vi "azcamtool.vi"() -> ()   [LabVIEW 2014]
doc: "AzCamTool"
uses:
  globals/AzCamGlobals.vi
  globals/DetectorGlobals.vi
panel:
  in  "Image Type":u16(ring) items=["zero", "object", "flat", "dark", "LED", "Fe55"]
  in  "Exposure Time":dbl=1.0 min=0.0 format="%<%S%3u>t"
  out "Image Filename":string
  out "StatusBar":string
  in  "TestImage":bool=TRUE caption="Test Image"
  in  "Image Title":string
  out "rowbin":u32=1 min=1 max=99 step=1
  out "colbin":u32=1 min=1 max=99 step=1
  out "progress":dbl(slide) scale=0.0..100.0 scale format="%.1e"
  out "CamTemp":sgl=-999.9 format="%.1f"
  out "DewTemp":sgl=-999.9 format="%.1f"
  out "SequenceCount":string caption="Seq. Count"
  out "Current Exposure Time":dbl caption="Exposure Time" min=0.0 format="%<%S%3u>t"
  out "ImageTypeName":string caption="ImageType"
  in  "Abort":bool
  in  "Reset":bool
  in  "Pause":bool
  in  "Resume":bool
  in  "Readout":bool
  out "CurrentImageTitle":string caption="ImageTitle"
  out "Error":bool
  in  "Expose":bool
  in  "Sequence":bool
  in  "Num Seq.":u16=1 min=1 step=1
  in  "Detector":bool
  in  "FilenameBut":bool caption="Filename"
  in  "Preferences":bool
  out "Test Image":bool
  # "Control"
  # "Status"
  # "Binning"
  # "Exposure Status"
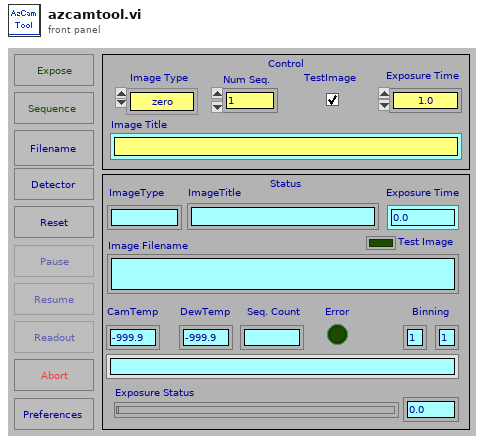
[diagram p1: front panel]
types:
  T1 = enum16{"Standard", "Buffered", "CRLF", "Immediate"}
  T2 = enum16{"Start", "Stop", "Abort", "Pause", "SetExposureTime", "GetExposureTimeRemaining", "Resume", "Readout", "GetExposureTime", "GetTotalPixels", "GetPixelsRemaining"}
  T3 = enum16{"Start", "Stop", "Abort", "Pause", "SetExposureTime", "GetExposureTimeRemaining", "Resume", "Readout", "GetExposureTime"}
  T4 = enum16{"Start", "Stop", "Abort", "Pause", "SetExposureTime", "GetExposureTimeRemaining", "Resume"}
  T5 = enum16{"Start", "Stop", "Abort", "Pause", "SetExposureTime", "GetExposureTimeRemaining", "Resume", "Readout"}
  T6 = enum32{"invalid app kind", "Development System", "Run Time System", "Student Edition", "Embedded LabVIEW", "Evaluation", "Custom"}
  T7 = enum32{"invalid OS target", "Mac OS", "Windows 3.1", "Windows 95/NT", "Solaris 1", "Solaris 2", "HP-UX", "PowerMAX", "Linux", "Irix", "Rhapsody", "BeOS", "AIX", "OSF1", "VxWorks", "PharLap", "Carbon", "RTX", "Windows x64", "Linux x64", "Mac OS X x64"}
  T8 = enum8{"Enabled", "Disabled", "Disabled and Grayed Out"}
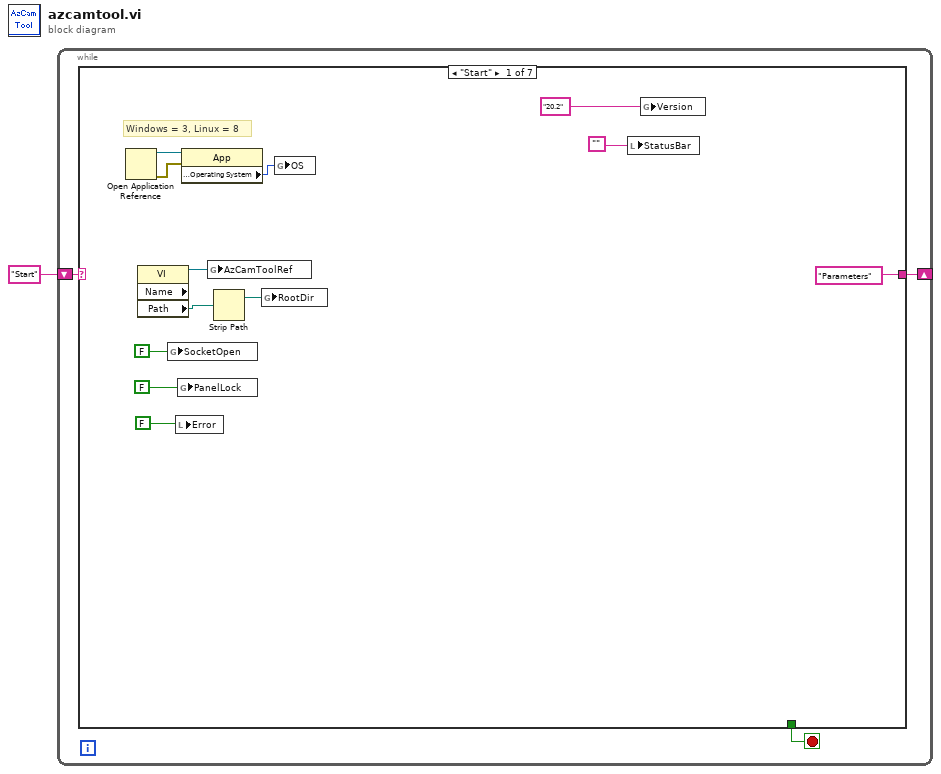
[diagram p0: block diagram]
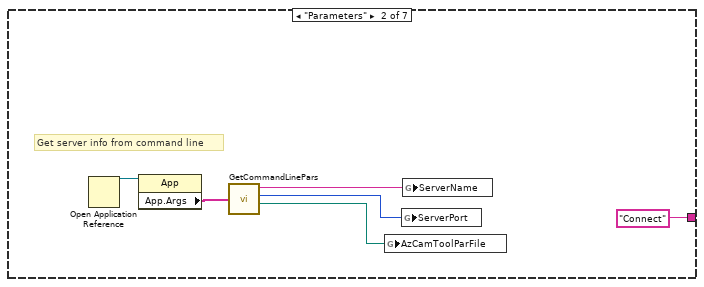
[diagram p2: hidden frame]
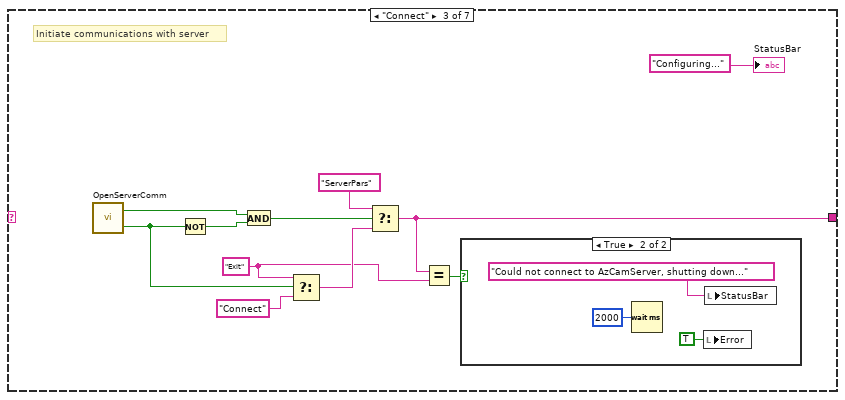
[diagram p3: hidden frame]
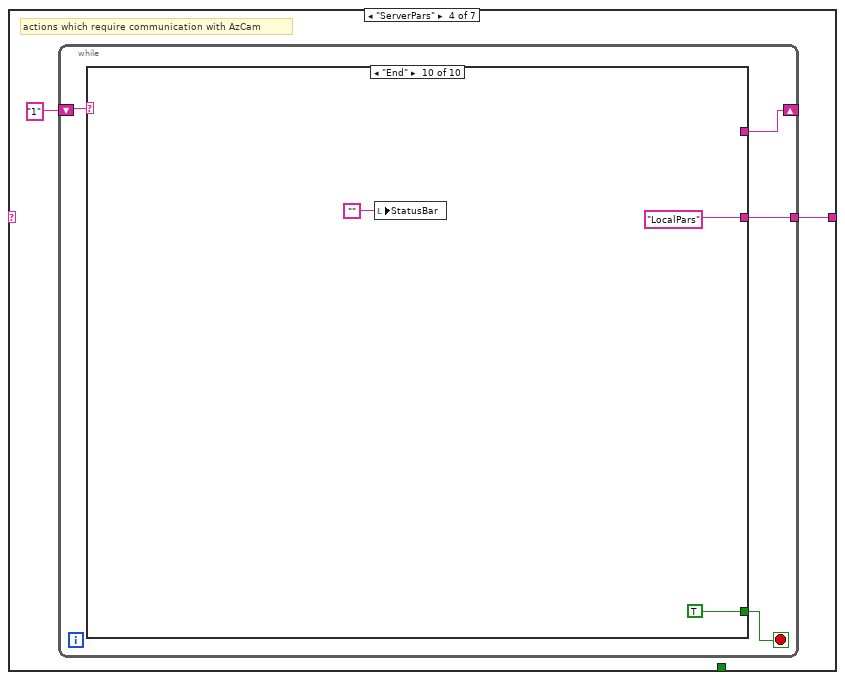
[diagram p5: hidden frame]
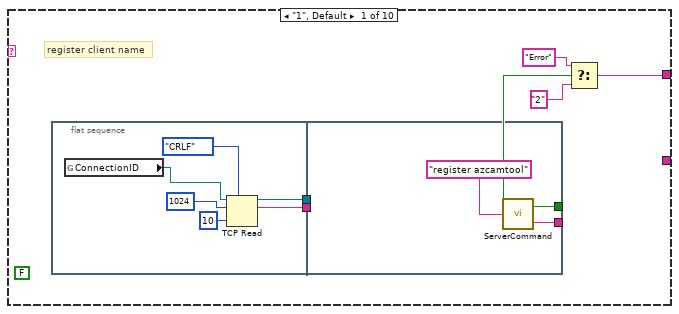
[diagram p6: hidden frame]
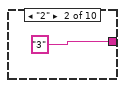
[diagram p7: hidden frame]
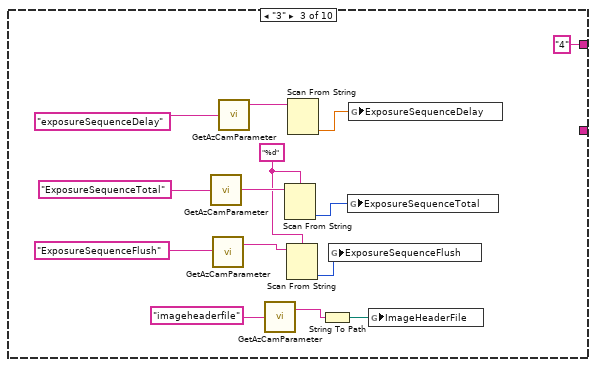
[diagram p8: hidden frame]
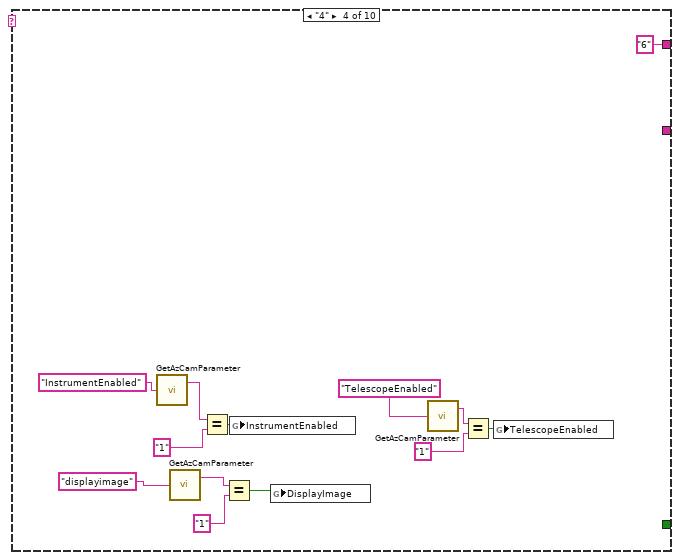
[diagram p9: hidden frame]
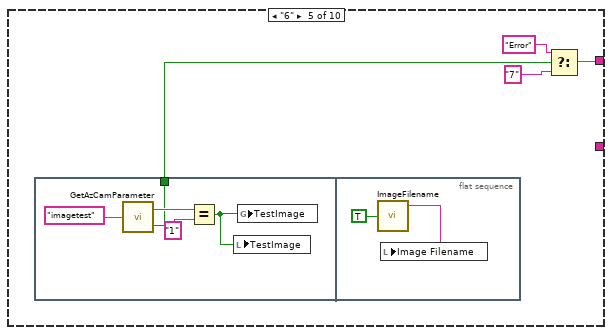
[diagram p10: hidden frame]
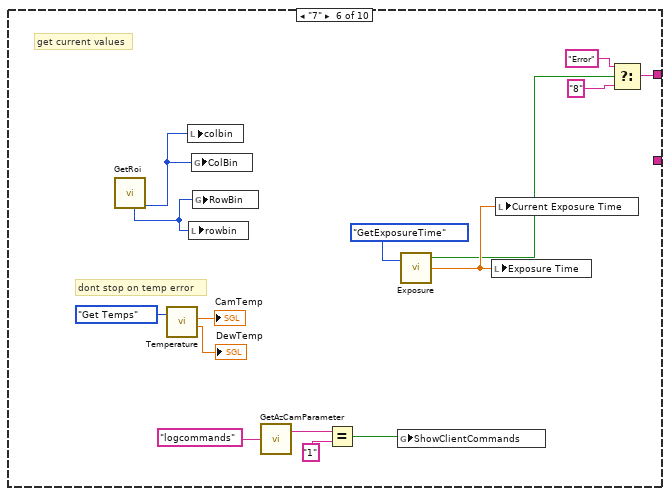
[diagram p11: hidden frame]
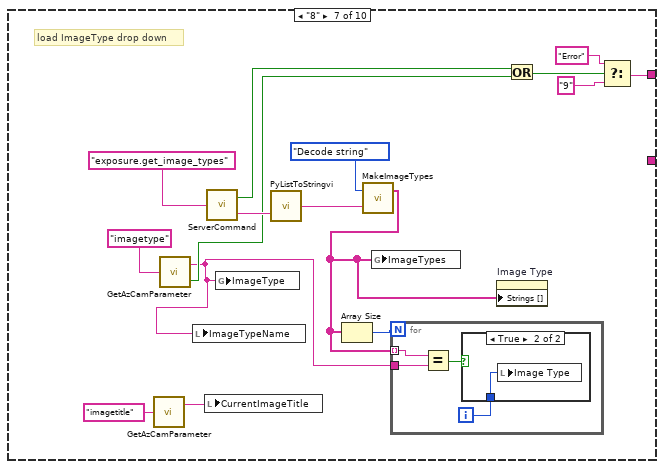
[diagram p12: hidden frame]
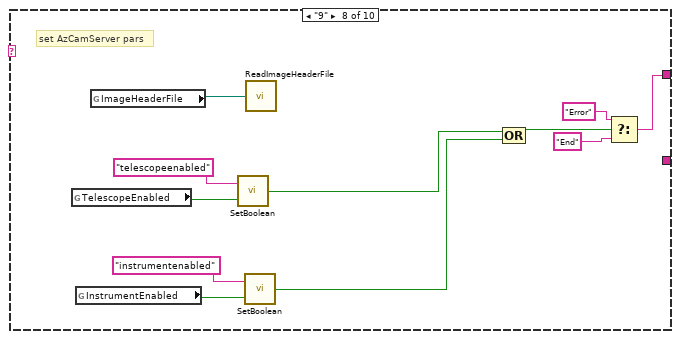
[diagram p14: hidden frame]
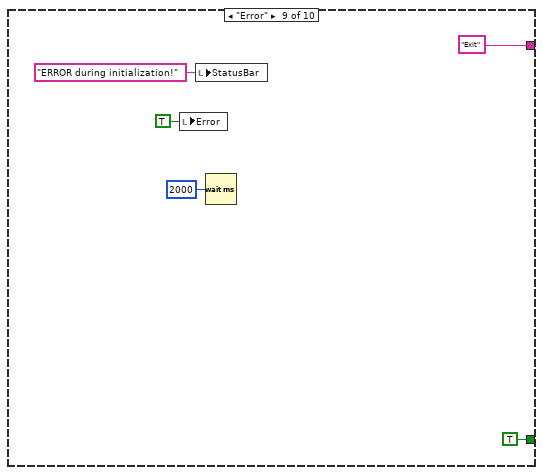
[diagram p15: hidden frame]
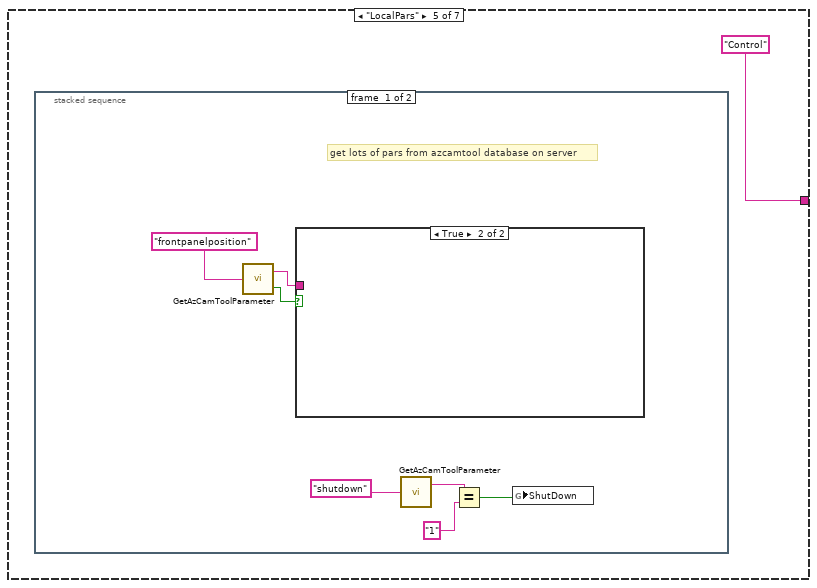
[diagram p16: hidden frame]
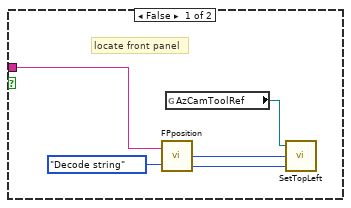
[diagram p17: hidden frame]
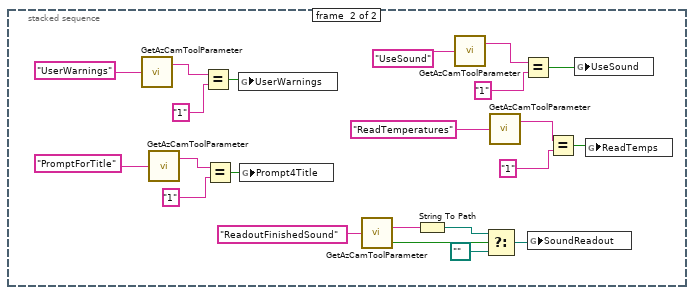
[diagram p18: hidden frame]
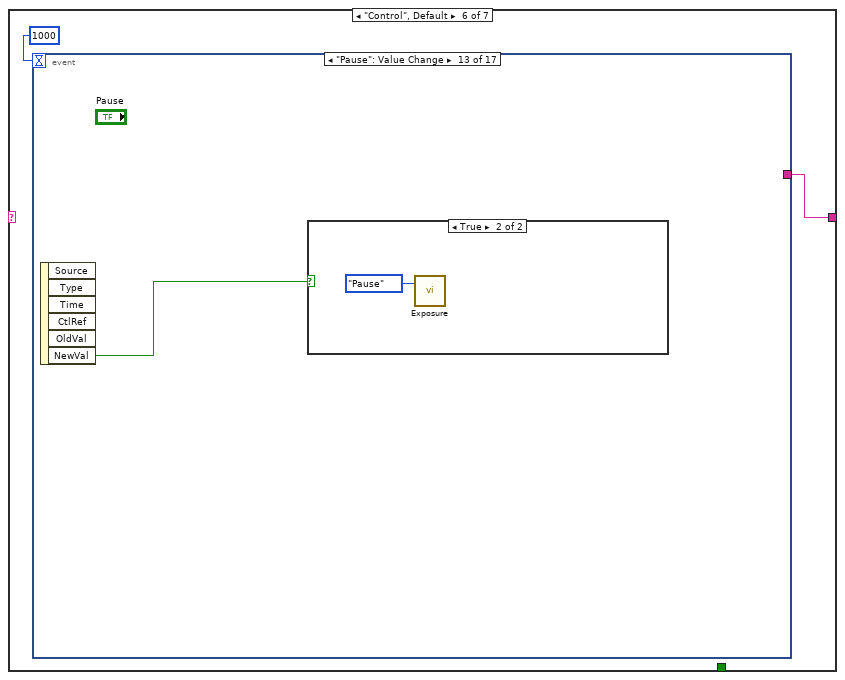
[diagram p19: hidden frame]
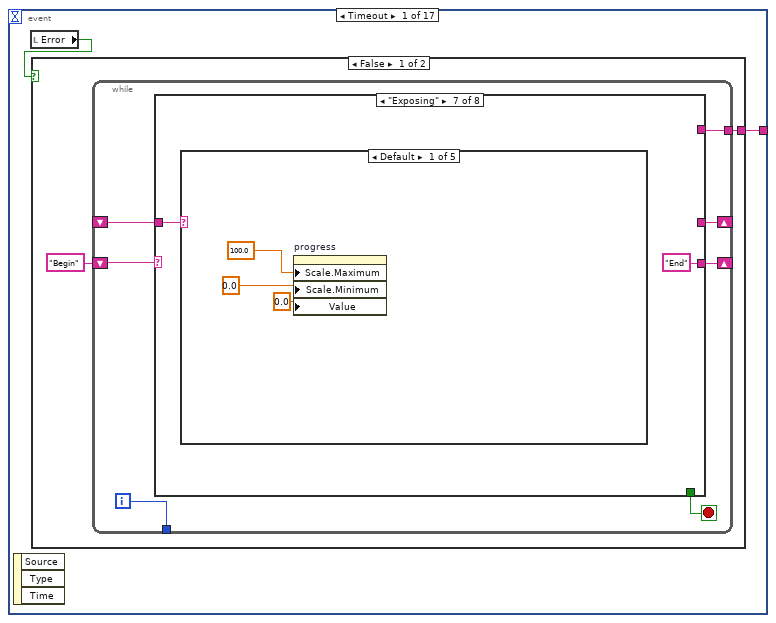
[diagram p20: hidden frame]
diagram:
  n1 = while {
    shift-right: [w2] -> _
    shift-left: "Start" ("Command") -> [w3]
    stop <- w4 stop-if-true
    n2 = case shown="\"Start\"" w3 {
      tunnel: [_ _ _ _ _ _ TRUE] -> w4
      tunnel: ["Parameters" "Connect" ("f") w25 w38 "Control" w188 _] -> w2
      frame "Start" {
        # "Windows = 3, Linux = 8"
        n3 = Open Application Reference() -> (0:w15:errorcluster, 3:w16:refnum<vi>)  [unwired: 4 in]
        n4 = property class="VI" props=["Name", "Path"]() -> (reference out=w7:refnum<vi>, "Path"=w11:path)  [unwired: 2 in, 2 out]
        n5 = global write "AzCamGlobals.vi" "SocketOpen"(FALSE ("SocketOpen")) -> ()
        n6 = local write "Error"(FALSE ("Error")) -> ()
        n7 = global write "AzCamGlobals.vi" "PanelLock"(FALSE ("LockFlag")) -> ()
        n8 = property class="App"(reference=w16, error in=w15) -> ("Application:Target:Operating System"=w13:T7)  [unwired: 2 out]
        n9 = global write "AzCamGlobals.vi" "AzCamToolRef"(w7) -> ()
        n10 = Strip Path(path=w11) -> (stripped path=w9:path)  [unwired: 1 out]
        n11 = global write "AzCamGlobals.vi" "RootDir"(w9) -> ()
        n12 = global write "AzCamGlobals.vi" "OS"(w13) -> ()
        n13 = local write "StatusBar"("") -> ()
        n14 = global write "AzCamGlobals.vi" "Version"("20.2" ("Version Date")) -> ()
      }
      frame "Parameters" {
        # "Get server info from command line"
        n15 = Open Application Reference() -> (3:w20:refnum<vi>)  [unwired: 4 in, 1 out]
        n16 = property class="App"(reference=w20) -> ("App.Args"=w21:string[])  [unwired: 1 in, 2 out]
        n17 = call "GetCommandLinePars.vi"("Command line array"=w21) -> ("Server"=w19:string, "Port"=w18:i32, "AzCamToolParFile"=w17:path)  [unwired: 1 out]
        n18 = global write "AzCamGlobals.vi" "AzCamToolParFile"(w17) -> ()
        n19 = global write "AzCamGlobals.vi" "ServerPort"(w18) -> ()
        n20 = global write "AzCamGlobals.vi" "ServerName"(w19) -> ()
      }
      frame "Connect" {
        w24 = "Exit" ("f")
        # "Initiate communications with server"
        n21 = call "OpenServerComm.vi"() -> ("Connected"=w32:bool, "Quitted"=w26:bool)  [unwired: 1 in]
        n22 = Not(x=w26) -> (.not. x?=w31:bool)
        n23 = And(x=w32, y=w31) -> (x .and. y?=w33:bool)
        n24 = Select(t=w24, s=w26, f="Connect") -> (s? t:f=w28:string)
        n25 = Select(t="ServerPars" ("f"), s=w33, f=w28) -> (s? t:f=w25:string)
        n26 = Equal?(x=w25, y=w24) -> (x = y?=w23:bool)
        n27 = case shown="True" w23 {
          frame False {
          }
          frame True {
            n28 = Wait (ms)(milliseconds to wait=u32 2000) -> ()  [unwired: 1 out]
            n29 = local write "Error"(TRUE ("Error")) -> ()
            n30 = local write "StatusBar"("Could not connect to AzCamServer, shutting down..." ("StatusBar")) -> ()
          }
        }
        "StatusBar" <- "Configuring..." ("Messages")
      }
      frame "ServerPars" {
        # "actions which require communication with AzCam"
        n31 = while {
          tunnel: [w40] -> w38
          shift-right: [w41] -> _
          shift-left: "1" ("key") -> [w42]
          stop <- w39 stop-if-true
          n32 = case shown="\"End\"" w42 {
            tunnel: [w46 "3" ("key") "4" ("key") "6" ("key") w87 w106 w118 w138 _ _] -> w41
            tunnel: [_ _ _ _ _ _ _ _ "Exit" "LocalPars"] -> w40
            tunnel: [_ _ _ _ _ _ _ _ TRUE TRUE] -> w39
            frame "1", Default {
              (unwired) FALSE
              # "register client name"
              n33 = flat-sequence {
                tunnel: [w51] -> w44
                tunnel: [w50] -> w43
                tunnel: [w56] -> _
                tunnel: [w55] -> w45
                tunnel: w44 -> [_]
                tunnel: w43 -> [_]
                frame #0 {
                  n34 = global read "AzCamGlobals.vi" "ConnectionID"() -> (w49:refnum<k5>)
                  n35 = TCP Read(connection ID=w49, bytes to read=1024, 7:T1."CRLF" ("mode (standard)"), 9:10 ("timeout ms (25000)")) -> (connection ID out=w50:refnum<k5>, data out=w51:string)  [unwired: 1 in, 1 out]
                }
                frame #1 {
                  n36 = call "ServerCommand.vi"("Command"="register azcamtool") -> ("Error"=w55:bool, "Reply"=w56:string)
                }
              }
              n37 = Select(t="Error" ("key"), s=w45, f="2" ("key")) -> (s? t:f=w46:string)
            }
            frame "2" {
            }
            frame "3" {
              w67 = "%d" ("format string")
              n38 = call "GetAzCamParameter.vi"("Parameter"="ExposureSequenceTotal") -> ("Value"=w71:string)  [unwired: 1 out]
              n39 = call "GetAzCamParameter.vi"("Parameter"="ExposureSequenceFlush") -> ("Value"=w62:string)  [unwired: 1 out]
              n40 = call "GetAzCamParameter.vi"("Parameter"="exposureSequenceDelay") -> ("Value"=w69:string)  [unwired: 1 out]
              n41 = call "GetAzCamParameter.vi"("Parameter"="imageheaderfile" ("key")) -> ("Value"=w61:string)  [unwired: 1 out]
              n42 = Scan From String(format string=w67, input string=w71) -> (output 1=w65:i32)  [unwired: 3 in, 3 out]
              n43 = Scan From String(format string=w67, input string=w62) -> (output 1=w66:i32)  [unwired: 3 in, 3 out]
              n44 = Scan From String(input string=w69) -> (output 1=w64:dbl)  [unwired: 4 in, 3 out]
              n45 = String To Path(string=w61) -> (path=w63:path)
              n46 = global write "AzCamGlobals.vi" "ExposureSequenceFlush"(w66) -> ()
              n47 = global write "AzCamGlobals.vi" "ExposureSequenceTotal"(w65) -> ()
              n48 = global write "AzCamGlobals.vi" "ExposureSequenceDelay"(w64) -> ()
              n49 = global write "AzCamGlobals.vi" "ImageHeaderFile"(w63) -> ()
            }
            frame "4" {
              n50 = call "GetAzCamParameter.vi"("Parameter"="InstrumentEnabled" ("key")) -> ("Value"=w73:string)  [unwired: 1 out]
              n51 = call "GetAzCamParameter.vi"("Parameter"="displayimage" ("key")) -> ("Value"=w76:string)  [unwired: 1 out]
              n52 = Equal?(x=w73, y="1") -> (x = y?=w81:bool)
              n53 = Equal?(x=w76, y="1") -> (x = y?=w80:bool)
              n54 = global write "AzCamGlobals.vi" "InstrumentEnabled"(w81) -> ()
              n55 = global write "AzCamGlobals.vi" "DisplayImage"(w80) -> ()
              n56 = call "GetAzCamParameter.vi"("Parameter"="TelescopeEnabled" ("key")) -> ("Value"=w77:string)  [unwired: 1 out]
              n57 = Equal?(x=w77, y="1") -> (x = y?=w84:bool)
              n58 = global write "AzCamGlobals.vi" "TelescopeEnabled"(w84) -> ()
            }
            frame "6" {
              n59 = flat-sequence {
                tunnel: [w90] -> w86
                frame #0 {
                  n60 = call "GetAzCamParameter.vi"("Parameter"="imagetest") -> ("Error"=w90:bool, "Value"=w91:string)
                  n61 = Equal?(x=w91, y="1") -> (x = y?=w94:bool)
                  n62 = local write "TestImage"(w94) -> ()
                  n63 = global write "AzCamGlobals.vi" "TestImage"(w94) -> ()
                }
                frame #1 {
                  n64 = call "ImageFilename.vi"("Immediate"=TRUE) -> ("Output Image Filename"=w96:string)  [unwired: 2 out]
                  n65 = local write "Image Filename"(w96) -> ()
                }
              }
              n66 = Select(t="Error" ("key"), s=w86, f="7" ("key")) -> (s? t:f=w87:string)
            }
            frame "7" {
              # "dont stop on temp error"
              # "get current values"
              n67 = call "GetRoi.vi"() -> ("RowBin"=w110:i32, "ColBin"=w111:i32)  [unwired: 1 in, 4 out]
              n68 = call "Temperature.vi"("Action"=enum16{"Set Celsius", "Get Temps"}."Get Temps") -> ("Output2"=→"DewTemp":sgl, "Output1"=→"CamTemp":sgl)  [unwired: 1 in, 3 out]
              n69 = local write "colbin"(w111) -> ()
              n70 = local write "rowbin"(w110) -> ()
              n71 = global write "DetectorGlobals.vi" "ColBin"(w111) -> ()
              n72 = global write "DetectorGlobals.vi" "RowBin"(w110) -> ()
              n73 = call "GetAzCamParameter.vi"("Parameter"="logcommands") -> ("Value"=w98:string)  [unwired: 1 out]
              n74 = Equal?(x=w98, y="1") -> (x = y?=w97:bool)
              n75 = global write "AzCamGlobals.vi" "ShowClientCommands"(w97) -> ()
              n76 = call "Exposure.vi"("Command"=T2."GetExposureTime") -> ("Error"=w101:bool, "float"=w102:dbl)  [unwired: 1 in, 1 out]
              n77 = local write "Exposure Time"(w102) -> ()
              n78 = local write "Current Exposure Time"(w102) -> ()
              n79 = Select(t="Error" ("key"), s=w101, f="8" ("key")) -> (s? t:f=w106:string)
            }
            frame "8" {
              # "load ImageType drop down"
              n80 = call "GetAzCamParameter.vi"("Parameter"="imagetitle") -> ("Value"=w112:string)  [unwired: 1 out]
              n81 = call "GetAzCamParameter.vi"("Parameter"="imagetype") -> ("Error"=w115:bool, "Value"=w114:string)
              n82 = local write "ImageTypeName"(w114) -> ()
              n83 = local write "CurrentImageTitle"(w112) -> ()
              n84 = call "ServerCommand.vi"("Command"="exposure.get_image_types") -> ("Error"=w116:bool, "Reply"=w125:string)
              n85 = global write "AzCamGlobals.vi" "ImageType"(w114) -> ()
              n86 = call "PyListToStringvi.vi"("PythonList"=w125) -> ("String"=w124:string)
              n87 = call "MakeImageTypes.vi"("String In"=w124, "Action"=enum16{"Make string", "Decode string"}."Decode string") -> ("ImageTypes"=w122:string[])  [unwired: 1 out]
              n88 = Array Size(array=w122) -> (size(s)=w123:i32)
              n89 = global write "AzCamGlobals.vi" "ImageTypes"(w122) -> ()
              n90 = for {
                N: w123 -> [_]
                tunnel: w122 -> [w131] mode=indexing
                tunnel: w114 -> [w130]
                i -> [w128]
                n91 = Equal?(x=w131, y=w130) -> (x = y?=w129:bool)
                n92 = case shown="True" w129 {
                  tunnel: w128 -> [_ w132]
                  frame False {
                  }
                  frame True {
                    n93 = local write "Image Type"(w132) -> ()
                  }
                }
              }
              n94 = property on="Image Type" class="Ring (strict)"("Strings []"=w122) -> ()  [unwired: 2 in, 2 out]
              n95 = Or(x=w116, y=w115) -> (x .or. y?=w117:bool)
              n96 = Select(t="Error" ("key"), s=w117, f="9" ("key")) -> (s? t:f=w118:string)
            }
            frame "9" {
              # "set AzCamServer pars"
              n97 = global read "AzCamGlobals.vi" "TelescopeEnabled"() -> (w135:bool)
              n98 = global read "AzCamGlobals.vi" "InstrumentEnabled"() -> (w134:bool)
              n99 = global read "AzCamGlobals.vi" "ImageHeaderFile"() -> (w133:path)
              n100 = call "SetBoolean.vi"("Boolean"=w135, "Attribute"="telescopeenabled" ("Command")) -> ("Error"=w137:bool)
              n101 = call "SetBoolean.vi"("Boolean"=w134, "Attribute"="instrumentenabled" ("Command")) -> ("Error"=w136:bool)
              n102 = call "ReadImageHeaderFile.vi"("ImageHeaderFile"=w133) -> ()  [unwired: 1 in]
              n103 = Compound Arithmetic op=OR(w137, w136) -> (w139:bool)
              n104 = Select(t="Error" ("key"), s=w139, f="End" ("key")) -> (s? t:f=w138:string)
            }
            frame "Error" {
              n105 = local write "Error"(TRUE ("Error")) -> ()
              n106 = local write "StatusBar"("ERROR during initialization!" ("StatusBar")) -> ()
              n107 = Wait (ms)(milliseconds to wait=u32 2000) -> ()  [unwired: 1 out]
            }
            frame "End" {
              n108 = local write "StatusBar"("") -> ()
            }
          }
        }
      }
      frame "LocalPars" {
        n109 = stacked-sequence {
          frame #0 {
            # "get lots of pars from azcamtool database on server"
            n110 = call "GetAzCamToolParameter.vi"("Parameter"="frontpanelposition" ("key")) -> ("Error"=w158:bool, "Value"=w159:string)
            n111 = case shown="True" w158 {
              tunnel: w159 -> [w160 _]
              frame False {
                # "locate front panel"
                n112 = call "FPposition.vi"("String In"=w160, "Action"=enum16{"Make string", "Decode string"}."Decode string") -> ("top"=w162:i32, "left"=w161:i32)  [unwired: 1 out]
                n113 = global read "AzCamGlobals.vi" "AzCamToolRef"() -> (w164:refnum<vi>)
                n114 = call "SetTopLeft.vi"("left"=w161, "top"=w162, "VI Ref"=w164) -> ()
              }
              frame True {
              }
            }
            n115 = call "GetAzCamToolParameter.vi"("Parameter"="shutdown" ("key")) -> ("Value"=w153:string)  [unwired: 1 out]
            n116 = Equal?(x=w153, y="1") -> (x = y?=w156:bool)
            n117 = global write "AzCamGlobals.vi" "ShutDown"(w156) -> ()
          }
          frame #1 {
            n118 = call "GetAzCamToolParameter.vi"("Parameter"="UserWarnings" ("key")) -> ("Value"=w167:string)  [unwired: 1 out]
            n119 = call "GetAzCamToolParameter.vi"("Parameter"="PromptForTitle" ("key")) -> ("Value"=w168:string)  [unwired: 1 out]
            n120 = Equal?(x=w167, y="1") -> (x = y?=w185:bool)
            n121 = Equal?(x=w168, y="1") -> (x = y?=w183:bool)
            n122 = global write "AzCamGlobals.vi" "UserWarnings"(w185) -> ()
            n123 = global write "AzCamGlobals.vi" "Prompt4Title"(w183) -> ()
            n124 = call "GetAzCamToolParameter.vi"("Parameter"="ReadoutFinishedSound" ("key")) -> ("Error"=w165:bool, "Value"=w169:string)
            n125 = String To Path(string=w169) -> (path=w177:path)
            n126 = call "GetAzCamToolParameter.vi"("Parameter"="UseSound" ("key")) -> ("Value"=w186:string)  [unwired: 1 out]
            n127 = Select(t=w177, s=w165, f=path "") -> (s? t:f=w179:path)
            n128 = call "GetAzCamToolParameter.vi"("Parameter"="ReadTemperatures" ("key")) -> ("Value"=w174:string)  [unwired: 1 out]
            n129 = Equal?(x=w186, y="1") -> (x = y?=w180:bool)
            n130 = global write "AzCamGlobals.vi" "SoundReadout"(w179) -> ()
            n131 = Equal?(x=w174, y="1") -> (x = y?=w176:bool)
            n132 = global write "AzCamGlobals.vi" "UseSound"(w180) -> ()
            n133 = global write "AzCamGlobals.vi" "ReadTemps"(w176) -> ()
          }
        }
      }
      frame "Control", Default {
        n134 = event shown="[12] \"Pause\": Value Change" {
          selector: _ -> [_ _ _ _ _ _ _ _ _ _ _ _ _ _ _ _ _]
          dyn-events: _ -> [_ _ _ _ _ _ _ _ _ _ _ _ _ _ _ _ _]
          timeout: 1000 -> [_ _ _ _ _ _ _ _ _ _ _ _ _ _ _ _ _]
          tunnel: [w190 "Control" ("Command") "Control" ("Command") _ _ _ _ _ _ _ _ _ _ _ _ "Exit" ("Command") w422] -> w188
          event Timeout {
            n135 = event-data() -> ()  [unwired: 1 in, 3 out]
            n136 = local read "Error"() -> (w189:bool)
            n137 = case shown="False" w189 {
              tunnel: [w191 w321] -> w190
              frame False {
                n138 = while {
                  shift-right: [w198] -> _
                  shift-left: "Begin" -> [w199]
                  tunnel: [w197] -> w191
                  tunnel: [w196] -> _
                  shift-right: [w195] -> _
                  shift-left: _ -> [w194]
                  i -> [w196]
                  stop <- w193 stop-if-true
                  n139 = case shown="\"Exposing\"" w199 {
                    tunnel: [w202 w213 "Pars" "TimeSync" "CheckExposing" w264 "End" _] -> w198
                    tunnel: [w200 _ _ w231 w253 w262 _ TRUE ("Error")] -> w193
                    tunnel: [w201 _ _ _ _ _ _ "Control"] -> w197
                    tunnel: [_ _ _ _ _ w267 _ _] -> w195
                    tunnel: w194 -> [_ _ _ _ _ _ w291 _]
                    frame "Begin", Default {
                      n140 = global read "AzCamGlobals.vi" "SocketOpen"() -> (w203:bool)
                      n141 = case shown="True" w203 {
                        tunnel: [_ "CheckErrorStatus"] -> w202
                        tunnel: ["Exit" ("f") _] -> w201
                        tunnel: [TRUE ("Quitted") FALSE ("Quitted")] -> w200
                        frame False {
                          n142 = local write "StatusBar"("No communication with AzCamServer... shutting down" ("message")) -> ()
                          n143 = Wait (ms)(milliseconds to wait=u32 1000) -> ()  [unwired: 1 out]
                        }
                        frame True {
                        }
                      }
                      n144 = local write "Error"(w200) -> ()
                    }
                    frame "CheckErrorStatus" {
                      n145 = call "GetAzCamParameter.vi"("Parameter"="errorstatus") -> ("Error"=w211:bool, "Value"=w210:string)
                      "Error" <- w211
                      n146 = case shown="False" w211 {
                        tunnel: w210 -> [_ w216]
                        tunnel: ["Temps" "End"] -> w213
                        frame False {
                          (unwired) FALSE ("Stop?")
                          # "no error"
                        }
                        frame True {
                          # "new - no popups"
                          n147 = local write "StatusBar"(w216) -> ()
                          n148 = Wait (ms)(milliseconds to wait=u32 2000) -> ()  [unwired: 1 out]
                        }
                      }
                    }
                    frame "Temps" {
                      # "update status on timeout only..."
                      n149 = flat-sequence {
                        frame #0 {
                          n150 = call "Temperature.vi"("Action"=enum16{"Set Celsius", "Get Temps"}."Get Temps") -> ("Output2"=w219:sgl, "Output1"=w220:sgl)  [unwired: 1 in, 3 out]
                          n151 = local write "CamTemp"(w220) -> ()
                          n152 = local write "DewTemp"(w219) -> ()
                        }
                        frame #1 {
                          n153 = call "GetAzCamParameter.vi"("Parameter"="imagetest" ("Attribute")) -> ("Value"=w224:string)  [unwired: 1 out]
                          n154 = Equal?(x=w224, y="1") -> (x = y?=→"Test Image":bool)
                          n155 = call "GetAzCamParameter.vi"("Parameter"="imagetitle" ("Attribute")) -> ("Value"=→"CurrentImageTitle":string)  [unwired: 1 out]
                        }
                      }
                    }
                    frame "Pars" {
                      n156 = call "GetBoolean.vi"("Attribute"="isexposuresequence") -> ("Error"=w230:bool, "Boolean"=w228:bool)
                      n157 = case shown="True" w228 {
                        tunnel: [_ w244] -> w233
                        tunnel: [_ w246] -> w232
                        tunnel: ["" w240] -> w229
                        frame False {
                        }
                        frame True {
                          n158 = call "GetAzCamParameter.vi"("Parameter"="exposuresequencenumber" ("Attribute")) -> ("Error"=w246:bool, "Value"=w243:string)
                          n159 = call "GetAzCamParameter.vi"("Parameter"="exposuresequencetotal" ("Attribute")) -> ("Error"=w244:bool, "Value"=w242:string)
                          n160 = Concatenate Strings(w243, "/" ("string"), w242) -> (w240:string)
                        }
                      }
                      "SequenceCount" <- w229
                      n161 = call "Exposure.vi"("Command"=T2."GetExposureTime") -> ("Error"=w234:bool, "float"=w236:dbl)  [unwired: 1 in, 1 out]
                      n162 = local write "Sequence"(w228) -> ()
                      n163 = case shown="False" w234 {
                        tunnel: w236 -> [w248 _]
                        frame False {
                          n164 = call "GetRoi.vi"() -> ("RowBin"=w250:i32, "ColBin"=w249:i32)  [unwired: 1 in, 4 out]
                          "rowbin" <- w250
                          "colbin" <- w249
                          n165 = global write "DetectorGlobals.vi" "ColBin"(w249) -> ()
                          n166 = global write "DetectorGlobals.vi" "RowBin"(w250) -> ()
                          "Current Exposure Time" <- w248
                        }
                        frame True {
                        }
                      }
                      n167 = Compound Arithmetic op=OR(w232, w233, w230, w234) -> (w231:bool)
                      n168 = local write "Error"(w231) -> ()
                    }
                    frame "TimeSync" {
                      n169 = call "GetBoolean.vi"("Attribute"="exposurecompleted") -> ("Error"=w253:bool, "Boolean"=w254:bool)
                      n170 = local write "Error"(w253) -> ()
                      n171 = call "ImageFilename.vi"("Immediate"=TRUE) -> ("Output Image Filename"=w252:string)  [unwired: 2 out]
                      n172 = case shown="True" w254 {
                        frame False {
                        }
                        frame True {
                          n173 = global read "AzCamGlobals.vi" "UseSound"() -> (w257:bool)
                          n174 = case shown="True" w257 {
                            frame False {
                            }
                            frame True {
                              n175 = global read "AzCamGlobals.vi" "SoundReadout"() -> (w258:path)
                              n176 = call "sound.vi"("Sound File"=w258) -> ()
                            }
                          }
                        }
                      }
                      n177 = local write "Image Filename"(w252) -> ()
                    }
                    frame "CheckExposing" {
                      n178 = call "GetAzCamParameter.vi"("Parameter"="exposureflag") -> ("Error"=w262:bool, "Value"=w261:string)
                      n179 = case shown="True" w262 {
                        tunnel: w261 -> [w287 _]
                        tunnel: [w285 w288] -> w268
                        tunnel: [w286 ""] -> w267
                        frame False {
                          n180 = call "ExposureStatusMessage.vi"("ExposureFlag"=w287) -> ("Message"=w286:string, "Exposing"=w285:bool)
                          n181 = local write "Expose"(w285) -> ()
                        }
                        frame True {
                          w288 = FALSE ("Exposing")
                          n182 = local write "Expose"(w288) -> ()
                        }
                      }
                      n183 = case shown="True" w268 {
                        tunnel: ["End" "Exposing"] -> w264
                        tunnel: w267 -> [_ w279]
                        tunnel: [w270 w282] -> w266
                        tunnel: [w270 w280] -> w265
                        frame False {
                          w270 = T8."Disabled and Grayed Out" ("Disabled")
                          n184 = local write "StatusBar"("") -> ()
                          n185 = local write "Pause"(FALSE ("Pause")) -> ()
                          "progress" <- 0.0 ("progress")
                        }
                        frame True {
                          w277 = T8."Enabled" ("Disabled")
                          w281 = T8."Disabled and Grayed Out" ("Disabled")
                          n186 = Equal?(x=w279, y="Exposure paused" ("Message")) -> (x = y?=w275:bool)
                          n187 = local write "StatusBar"(w279) -> ()
                          n188 = Equal?(x=w279, y="Reading image" ("Message")) -> (x = y?=w276:bool)
                          n189 = Or(x=w275, y=w276) -> (x .or. y?=w274:bool)
                          n190 = Select(t=w277, s=w275, f=w281) -> (s? t:f=w282:T8)
                          n191 = Select(t=w281, s=w274, f=w277) -> (s? t:f=w280:T8)
                        }
                      }
                      n192 = property on="Readout" class="Bool"("DisabledEnum"=w266) -> ()  [unwired: 2 in, 2 out]
                      n193 = property on="Resume" class="Bool"("DisabledEnum"=w266) -> ()  [unwired: 2 in, 2 out]
                      n194 = property on="Pause" class="Bool (strict)"("DisabledEnum"=w265) -> ()  [unwired: 2 in, 2 out]
                      n195 = call "GetAzCamParameter.vi"("Parameter"="imagetype") -> ("Value"=→"ImageTypeName":string)  [unwired: 1 out]
                      n196 = local write "Error"(w262) -> ()
                    }
                    frame "Exposing" {
                      n197 = case shown="Default" w291 {
                        selector: w291 -> [_ w299 w305 w314 w317]
                        frame Default {
                          n198 = property on="progress" class="Slide (strict)"("Scale.Maximum"=100.0 ("Scale.Range:Maximum"), "Scale.Minimum"=0.0 ("Scale.Range:Minimum"), "Value"=0.0 ("progress")) -> ()  [unwired: 2 in, 2 out]
                        }
                        frame "Exposing" {
                          n199 = local write "StatusBar"(w299) -> ()
                          n200 = call "Exposure.vi"("Command"=T3."GetExposureTimeRemaining") -> ("float"=w297:dbl)  [unwired: 1 in, 2 out]
                          n201 = call "Exposure.vi"("Command"=T2."GetExposureTime") -> ("float"=w295:dbl)  [unwired: 1 in, 2 out]
                          n202 = property on="progress" class="Slide (strict)"("Scale.Maximum"=w295, "Scale.Minimum"=0.0 ("Scale.Range:Minimum"), "Value"=w297) -> ()  [unwired: 2 in, 2 out]
                        }
                        frame "Exposure paused" {
                          n203 = local write "StatusBar"(w305) -> ()
                          n204 = call "Exposure.vi"("Command"=T3."GetExposureTimeRemaining") -> ("float"=w303:dbl)  [unwired: 1 in, 2 out]
                          n205 = call "Exposure.vi"("Command"=T2."GetExposureTime") -> ("float"=w301:dbl)  [unwired: 1 in, 2 out]
                          n206 = property on="progress" class="Slide (strict)"("Scale.Maximum"=w301, "Scale.Minimum"=0.0 ("Scale.Range:Minimum"), "Value"=w303) -> ()  [unwired: 2 in, 2 out]
                        }
                        frame "Reading image" {
                          n207 = local write "StatusBar"(w314) -> ()
                          n208 = call "Exposure.vi"("Command"=T2."GetTotalPixels") -> ("integer"=w307:i32)  [unwired: 1 in, 2 out]
                          n209 = call "Exposure.vi"("Command"=T2."GetPixelsRemaining") -> ("integer"=w310:i32)  [unwired: 1 in, 2 out]
                          n210 = Divide(x=w310, y=w307) -> (x/y=w313:dbl)
                          n211 = Multiply(x=w313, y=100.0) -> (x*y=w309:dbl)
                          n212 = property on="progress" class="Slide (strict)"("Scale.Maximum"=100.0 ("Scale.Range:Maximum"), "Scale.Minimum"=0.0 ("Scale.Range:Minimum"), "Value"=w309) -> ()  [unwired: 2 in, 2 out]
                        }
                        frame "Image Writing" {
                          n213 = local write "StatusBar"(w317) -> ()
                          n214 = local write "progress"(0.0 ("progress")) -> ()
                        }
                      }
                    }
                    frame "End" {
                    }
                  }
                }
              }
              frame True {
                # "pause to see error message then clear"
                n215 = local read "StatusBar"() -> (w322:string)
                n216 = String Length(string=w322) -> (length=w327:i32)
                n217 = Equal To 0?(x=w327) -> (x = 0?=w323:bool)
                n218 = flat-sequence {
                  tunnel: w324 -> [w328]
                  tunnel: ["Control" ("f")] -> w321
                  frame #0 {
                    n219 = Wait (ms)(milliseconds to wait=w328) -> ()  [unwired: 1 out]
                  }
                  frame #1 {
                    n220 = local write "StatusBar"("" ("StatusBar")) -> ()
                    n221 = local write "Error"(FALSE ("Error")) -> ()
                  }
                }
                n222 = Select(t=u32 0 ("milliseconds to wait"), s=w323, f=u32 2000 ("milliseconds to wait")) -> (s? t:f=w324:u32)
              }
            }
          }
          event "Expose": Value Change {
            # "start exposure process"
            n223 = event-data() -> ("NewVal"=w333:bool)  [unwired: 1 in, 4 out]
            n224 = case shown="True" w333 {
              frame False {
              }
              frame True {
                n225 = local read "Exposure Time"() -> (w343:dbl)
                n226 = property on="Image Type" class="Ring (strict)"() -> ("RingText.Text"=w338:string)  [unwired: 2 in, 2 out]
                n227 = local read "Image Title"() -> (w335:string)
                n228 = Format Into String(format string="%.03f", w343) -> (resulting string=w339:string)  [unwired: 2 in, 1 out]
                n229 = call "Quoter.vi"("String In"=w335) -> ("String Out"=w334:string)
                n230 = call "Exposure.vi"("Command"=T2."GetTotalPixels") -> ("integer"=w336:i32)  [unwired: 1 in, 2 out]
                n231 = global write "AzCamGlobals.vi" "TotalPixels"(w336) -> ()
                n232 = call <vilib>:"Space Constant.vi"() -> ("String"=w341:string)
                n233 = Concatenate Strings("exposure.expose1", w341, w339, w341, w338, w341, w334) -> (w340:string)
                n234 = call "ServerCommand.vi"("Command"=w340) -> ()  [unwired: 2 out]
              }
            }
          }
          event "Sequence": Value Change {
            n235 = event-data() -> ("OldVal"=w346:bool, "NewVal"=w345:bool)  [unwired: 1 in, 4 out]
            n236 = local read "Expose"() -> (w349:bool)
            n237 = Not(x=w349) -> (.not. x?=w348:bool)
            n238 = Compound Arithmetic op=AND(w345, w348) -> (w350:bool)
            n239 = case shown="True" w350 {
              tunnel: w346 -> [w352 _]
              tunnel: w345 -> [w354 _]
              frame False {
                n240 = Not(x=w354) -> (.not. x?=w353:bool)
                n241 = Compound Arithmetic op=AND(w352, w353) -> (w351:bool)
                n242 = case shown="True" w351 {
                  frame False {
                  }
                  frame True {
                    n243 = stacked-sequence {
                      frame #0 {
                        n244 = local write "StatusBar"("stopping exposure sequence..." ("StatusBar")) -> ()
                      }
                      frame #1 {
                        n245 = call "SetAzCamParameter.vi"("Value"="0", "Parameter"="isexposuresequence" ("Command")) -> ()  [unwired: 1 out]
                        n246 = call "SetAzCamParameter.vi"("Value"="1", "Parameter"="exposuresequencetotal" ("Attribute")) -> ()  [unwired: 1 out]
                      }
                    }
                  }
                }
              }
              frame True {
                n247 = local read "Test Image"() -> (w361:bool)
                n248 = global read "AzCamGlobals.vi" "UserWarnings"() -> (w362:bool)
                n249 = And(x=w362, y=w361) -> (x .and. y?=w360:bool)
                n250 = case shown="True" w360 {
                  tunnel: [TRUE ("T button?") w365] -> w363
                  frame False {
                  }
                  frame True {
                    n251 = Two Button Dialog(message="Do you really want to take a sequence of test exposures?", 2:"Yes" ("button name (\"OK\")")) -> (T button?=w365:bool)  [unwired: 1 in]
                  }
                }
                n252 = case shown="True" w363 {
                  frame False {
                  }
                  frame True {
                    n253 = stacked-sequence {
                      frame #0 {
                        n254 = local read "Exposure Time"() -> (w368:dbl)
                        n255 = call "Exposure.vi"("Command"=T2."SetExposureTime", "Exposure Time"=w368) -> ()  [unwired: 3 out]
                      }
                      frame #1 {
                        n256 = property on="Image Type" class="Ring (strict)"() -> ("RingText.Text"=w370:string)  [unwired: 2 in, 2 out]
                        n257 = call "ImageType.vi"("ImageType"=w370) -> ()  [unwired: 4 out]
                      }
                      frame #2 {
                        n258 = global read "AzCamGlobals.vi" "ExposureSequenceDelay"() -> (w371:dbl)
                        n259 = Format Into String(w371) -> (resulting string=w373:string)  [unwired: 3 in, 1 out]
                        n260 = call "SetAzCamParameter.vi"("Value"=w373, "Parameter"="exposuresequencedelay" ("string")) -> ()  [unwired: 1 out]
                      }
                      frame #3 {
                        n261 = call "Exposure.vi"("Command"=T2."GetTotalPixels") -> ("integer"=w374:i32)  [unwired: 1 in, 2 out]
                        n262 = global write "AzCamGlobals.vi" "TotalPixels"(w374) -> ()
                      }
                      frame #4 {
                        n263 = Format Into String("Num Seq.") -> (resulting string=w379:string)  [unwired: 3 in, 1 out]
                        n264 = call <vilib>:"Space Constant.vi"() -> ("String"=w377:string)
                        n265 = Concatenate Strings("exposure.sequence1 " ("Command"), w379, w377, "-1") -> (w378:string)
                        n266 = call "ServerCommand.vi"("Command"=w378) -> ()  [unwired: 2 out]
                      }
                    }
                  }
                }
              }
            }
          }
          event "Detector": Value Change {
            n267 = event-data() -> ()  [unwired: 1 in, 6 out]
            n268 = flat-sequence {
              frame #0 {
                n269 = call "DetPars.vi"("Immediate"=FALSE) -> ()  [unwired: 1 out]
              }
              frame #1 {
                n270 = global read "DetectorGlobals.vi" "ColBin"() -> (w384:i32)
                n271 = global read "DetectorGlobals.vi" "RowBin"() -> (w383:i32)
                n272 = local write "rowbin"(w383) -> ()
                n273 = local write "colbin"(w384) -> ()
              }
              frame #2 {
              }
              frame #3 {
                n274 = call "SavePars.vi"() -> ()  [unwired: 1 in, 1 out]
              }
            }
          }
          event "Preferences": Value Change {
            n275 = event-data() -> ()  [unwired: 1 in, 6 out]
            n276 = stacked-sequence {
              frame #0 {
                n277 = call "Preferences.vi"() -> ()  [unwired: 1 in]
              }
              frame #1 {
                n278 = call "SavePars.vi"() -> ()  [unwired: 1 in, 1 out]
              }
            }
          }
          event "Reset": Value Change {
            n279 = event-data() -> ()  [unwired: 1 in, 5 out]
            n280 = flat-sequence {
              frame #0 {
                n281 = call "ResetController.vi"() -> ()  [unwired: 2 in, 1 out]
              }
              frame #1 {
              }
            }
          }
          event "FilenameBut": Value Change {
            n282 = event-data() -> ()  [unwired: 1 in, 5 out]
            n283 = flat-sequence {
              frame #0 {
                n284 = call "ImageFilename.vi"("Immediate"=FALSE) -> ("Output Image Filename"=w386:string, "TestImage"=w388:bool, "Error"=w385:bool)
                n285 = case shown="False" w385 {
                  tunnel: w388 -> [w390 _]
                  tunnel: w386 -> [w389 _]
                  frame False {
                    n286 = local write "TestImage"(w390) -> ()
                    n287 = call "SavePars.vi"() -> ()  [unwired: 1 in, 1 out]
                    "Image Filename" <- w389
                  }
                  frame True {
                  }
                }
              }
              frame #1 {
              }
            }
          }
          event "TestImage": Value Change {
            n288 = event-data() -> ()  [unwired: 1 in, 6 out]
            n289 = flat-sequence {
              frame #0 {
                n290 = Select(t="1", s="TestImage", f="0") -> (s? t:f=w391:string)
                n291 = global write "AzCamGlobals.vi" "TestImage"("TestImage") -> ()
                n292 = call "SetAzCamParameter.vi"("Value"=w391, "Parameter"="imagetest") -> ()  [unwired: 1 out]
              }
              frame #1 {
                n293 = call "ImageFilename.vi"("Immediate"=TRUE) -> ("Output Image Filename"=w397:string)  [unwired: 2 out]
                n294 = local write "Image Filename"(w397) -> ()
              }
            }
          }
          event "Image Type": Value Change {
            n295 = event-data() -> ()  [unwired: 1 in, 6 out]
            n296 = property on="Image Type" class="Ring (strict)"() -> ("RingText.Text"=w398:string)  [unwired: 2 in, 2 out]
            n297 = call "ImageType.vi"("ImageType"=w398) -> ()  [unwired: 4 out]
          }
          event "Image Title": Value Change {
            n298 = event-data() -> ()  [unwired: 1 in, 6 out]
            n299 = call "Quoter.vi"("String In"="Image Title") -> ("String Out"=w399:string)
            n300 = call "SetAzCamParameter.vi"("Value"=w399, "Parameter"="imagetitle ") -> ()  [unwired: 1 out]
          }
          event "Exposure Time": Value Change {
            n301 = event-data() -> ("NewVal"=w403:dbl)  [unwired: 1 in, 5 out]
            n302 = call "Exposure.vi"("Command"=T2."SetExposureTime", "Exposure Time"=w403) -> ()  [unwired: 3 out]
          }
          event "Abort": Value Change {
            n303 = event-data() -> ()  [unwired: 1 in, 6 out]
            n304 = call "Exposure.vi"("Command"=T2."Abort") -> ("Error"=w404:bool)  [unwired: 1 in, 2 out]
            n305 = stacked-sequence {
              tunnel: w404 -> [_]
              frame #0 {
                n306 = local read "Sequence"() -> (w407:bool)
                n307 = local write "Abort"(FALSE ("Abort")) -> ()
                n308 = case shown="True" w407 {
                  frame False {
                    n309 = local write "progress"(0.0 ("progress")) -> ()
                  }
                  frame True {
                    n310 = Wait (ms)(milliseconds to wait=u32 1000) -> ()  [unwired: 1 out]
                    n311 = local write "StatusBar"("aborting sequence and current exposure" ("StatusBar")) -> ()
                  }
                }
              }
            }
          }
          event "Pause": Value Change {
            n312 = event-data() -> ("NewVal"=w411:bool)  [unwired: 1 in, 5 out]
            n313 = case shown="True" w411 {
              frame False {
              }
              frame True {
                n314 = call "Exposure.vi"("Command"=T4."Pause") -> ()  [unwired: 1 in, 3 out]
              }
            }
          }
          event "Readout": Value Change {
            n315 = event-data() -> ()  [unwired: 1 in, 6 out]
            n316 = call "Exposure.vi"("Command"=T5."Readout") -> ()  [unwired: 1 in, 3 out]
          }
          event "Resume": Value Change {
            n317 = event-data() -> ()  [unwired: 1 in, 6 out]
            n318 = call "Exposure.vi"("Command"=T5."Resume") -> ("Error"=w414:bool)  [unwired: 1 in, 2 out]
            n319 = stacked-sequence {
              tunnel: w414 -> [_]
              frame #0 {
                n320 = local write "Pause"(FALSE ("Pause")) -> ()
              }
            }
          }
          event Panel Close {
            n321 = event-data() -> ()  [unwired: 1 in, 4 out]
            n322 = One Button Dialog(message="close") -> ()  [unwired: 1 in, 1 out]
          }
          event Menu Selection (User) {
            n323 = event-data() -> ("MenuRef"=w421:refnum<k9>, "ItemTag"=w420:string, "ItemPath"=w419:string)  [unwired: 1 in, 4 out]
            n324 = call "MenuFind.vi"("TagIn"=w419) -> ("Menu"=w423:string)
            n325 = case shown="\"File\"" w423 {
              tunnel: w421 -> [_ _ w427]
              tunnel: [_ w425 _] -> w422
              tunnel: w420 -> [_ w424 w428]
              frame Default {
              }
              frame "File" {
                n326 = case shown="\"Exit\"" w424 {
                  tunnel: [_ "Exit" ("Command")] -> w425
                  frame Default {
                  }
                  frame "Exit" {
                  }
                }
              }
              frame "Help" {
                n327 = case shown="\"DisplayTips\"" w428 {
                  selector: w428 -> [_ w431 _]
                  tunnel: w427 -> [_ w429 _]
                  frame Default {
                  }
                  frame "DisplayTips" {
                    n328 = call "MenuToggle.vi"("item tag"=w431, "menubar"=w429) -> ("checked"=w430:bool)
                    n329 = property class="App"("Application:Show FP Tip Strips"=w430) -> ()  [unwired: 2 in, 2 out]
                  }
                  frame "AboutAzCam" {
                    w433 = "Written by Michael Lesser, University of Arizona\nSend comments to lesser@itl.arizona.edu\nSee http://www.itl.arizona.edu\n© 2013 Arizona Board of Regents. All rights reserved.\nLabVIEW is copyright National Instruments, Inc."  # Written by Michael Lesser, University of Arizona Send comments to lesser@itl.arizona.edu See http://www.itl.arizona.edu © 2013 Arizona Board of Regents. All rights reserved. LabVIEW is copyright National Instruments, Inc.
                    n330 = global read "AzCamGlobals.vi" "Version"() -> (w435:string)
                    n331 = Concatenate Strings("Version: " ("message"), w435, w433) -> (w432:string)
                    n332 = One Button Dialog(message=w432) -> ()  [unwired: 1 in, 1 out]
                  }
                }
              }
            }
          }
        }
      }
      frame "Exit" {
        n333 = stacked-sequence {
          frame #0 {
            # "update ConfigFile"
            n334 = stacked-sequence {
              frame #0 {
                n335 = call "FPposition.vi"("Action"=enum16{"Make string", "Decode string"}."Make string") -> ("String Out"=w439:string)  [unwired: 1 in, 2 out]
                n336 = call "SetAzCamToolParameter.vi"("Value"=w439, "Parameter"="frontpanelposition" ("key")) -> ()  [unwired: 1 out]
              }
              frame #1 {
                n337 = global read "AzCamGlobals.vi" "UserWarnings"() -> (w442:bool)
                n338 = Select(t="1" ("y"), s=w442, f="0" ("y")) -> (s? t:f=w440:string)
                n339 = call "SetAzCamToolParameter.vi"("Value"=w440, "Parameter"="UserWarnings" ("key")) -> ()  [unwired: 1 out]
              }
              frame #2 {
                n340 = global read "AzCamGlobals.vi" "Prompt4Title"() -> (w449:bool)
                n341 = Select(t="1" ("y"), s=w449, f="0" ("y")) -> (s? t:f=w445:string)
                n342 = call "SetAzCamToolParameter.vi"("Value"=w445, "Parameter"="PromptForTitle" ("key")) -> ()  [unwired: 1 out]
              }
              frame #3 {
                n343 = global read "AzCamGlobals.vi" "UseSound"() -> (w459:bool)
                n344 = Select(t="1" ("Parameter"), s=w459, f="0" ("Parameter")) -> (s? t:f=w452:string)
                n345 = global read "AzCamGlobals.vi" "ReadTemps"() -> (w454:bool)
                n346 = call "SetAzCamToolParameter.vi"("Value"=w452, "Parameter"="UseSound") -> ()  [unwired: 1 out]
                n347 = Select(t="1" ("Parameter"), s=w454, f="0" ("Parameter")) -> (s? t:f=w450:string)
                n348 = call "SetAzCamToolParameter.vi"("Value"=w450, "Parameter"="ReadTemperatures") -> ()  [unwired: 1 out]
              }
              frame #4 {
                n349 = call "SavePars.vi"() -> ()  [unwired: 1 in, 1 out]
              }
            }
          }
          frame #1 {
            n350 = flat-sequence {
              frame #0 {
                n351 = global read "AzCamGlobals.vi" "ShutDown"() -> (w460:bool)
                n352 = case shown="True" w460 {
                  frame False {
                  }
                  frame True {
                    n353 = call "ServerCommand.vi"("Command"="exitazcam") -> ()  [unwired: 2 out]
                  }
                }
              }
              frame #1 {
                n354 = global write "AzCamGlobals.vi" "SocketOpen"(FALSE ("SocketOpen?")) -> ()
                n355 = global read "AzCamGlobals.vi" "ConnectionID"() -> (w463:refnum<k5>)
                n356 = TCP Close Connection(connection ID=w463) -> ()  [unwired: 2 in, 2 out]
              }
            }
          }
          frame #2 {
            # "close AzCamTool"
            n357 = property class="App"() -> ("Application:Kind"=w466:T6)  [unwired: 2 in, 2 out]
            n358 = Equal?(x=w466, y=T6."Run Time System" ("Application:Kind")) -> (x = y?=w464:bool)
            n359 = case shown="False" w464 {
              selector: w464 -> [_ w467]
              frame False {
                n360 = Stop() -> ()  [unwired: 1 in]
              }
              frame True {
                n361 = Quit LabVIEW(quit? (T)=w467) -> ()
              }
            }
          }
        }
      }
    }
  }
